vi "Create New Class or Interface in Library.vi"(6 "directory (empty)":path, 8 "error in":errorcluster, 9 "create interface":bool, 10 "new class file name":string, 11 "library reference in":refnum<vi>) -> (0 "error out":errorcluster, 2 "class reference":refnum<vi>, 3 "library reference out":refnum<vi>)   [LabVIEW 2020]
doc: "Creates a new class or interface in memory. The new class or interface is not saved to disk even if you supply a <b>directory</b>. The <b>directory</b> specifies an initial location for the class should you choose to save it to disk later. If you specify an empty directory, then the new class or interface will be assigned an initial path relative to its owning library (if any), the the current project (if any) or the LabVIEW Data directory."
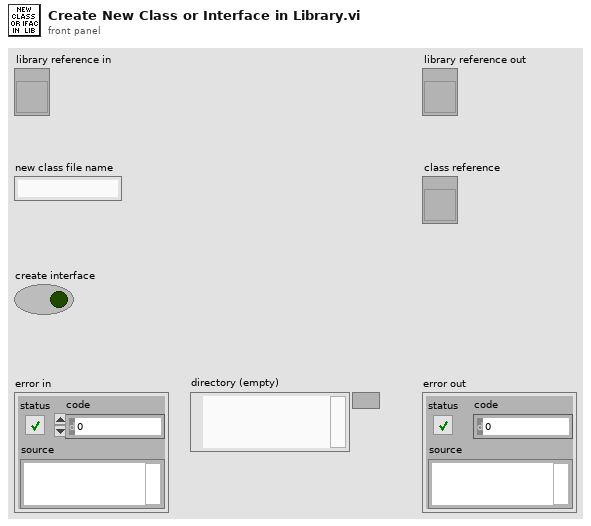
[diagram p1: front panel]
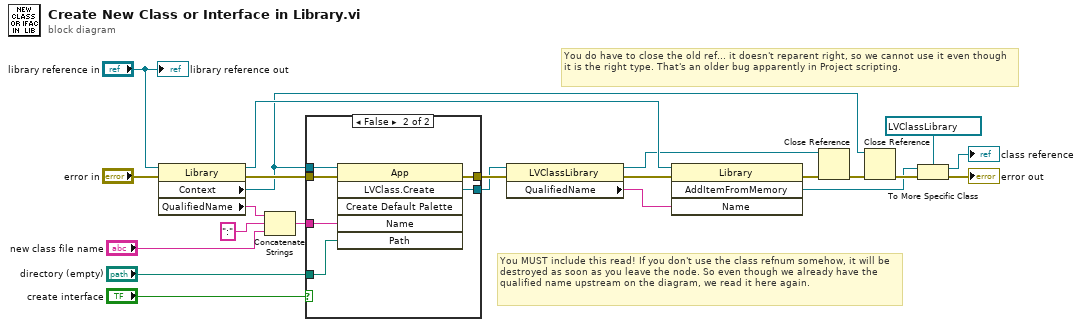
[diagram p0: block diagram]
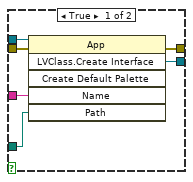
[diagram p2: hidden frame]
diagram:
  # "You do have to close the old ref... it doesn't reparent right, so we cannot use it even though it is the right type. That's an older bug apparently in Project scripting."
  # "You MUST include this read! If you don't use the class refnum somehow, it will be destroyed as soon as you leave the node. So even though we already have the qualified name upstream on the diagram, we read it here again."
  n1 = property class="Library"(reference="library reference in", error in="error in") -> (reference out=w14:refnum<vi>, error out=w23:errorcluster, "Context"=w2:refnum<vi>, "QualifiedName"=w13:string)
  n2 = Concatenate Strings(w13, ":" ("Name"), "new class file name") -> (w3:string)
  n3 = case shown="False" "create interface" {
    tunnel: w23 -> [w29 w35]
    tunnel: w3 -> [w27 w33]
    tunnel: [w26 w32] -> w12
    tunnel: [w28 w34] -> w22
    tunnel: w2 -> [w25 w30]
    tunnel: "directory (empty)" -> [w24 w31]
    frame True {
      n4 = invoke class="App" method="LVClass.Create Interface"(reference=w25, error in=w29, "Name"=w27, "Path"=w24) -> (error out=w28:errorcluster, "LVClass.Create Interface"=w26:refnum<vi>)  [unwired: 2 in, 4 out]
    }
    frame False {
      n5 = invoke class="App" method="LVClass.Create"(reference=w30, error in=w35, "Name"=w33, "Path"=w31) -> (error out=w34:errorcluster, "LVClass.Create"=w32:refnum<vi>)  [unwired: 2 in, 4 out]
    }
  }
  n6 = property class="LVClassLibrary"(reference=w12, error in=w22) -> (reference out=w10:refnum<vi>, error out=w21:errorcluster, "QualifiedName"=w1:string)
  n7 = invoke class="Library" method="AddItemFromMemory"(reference=w14, error in=w21, "Name"=w1) -> (error out=w19:errorcluster, "AddItemFromMemory"=w11:refnum<vi>)  [unwired: 1 in, 2 out]
  n8 = Close Reference(reference=w10, error in (no error)=w19) -> (error out=w17:errorcluster)
  n9 = Close Reference(reference=w2, error in (no error)=w17) -> (error out=w16:errorcluster)
  n10 = To More Specific Class(target class=refnum<vi> refnum ("reference out"), reference=w11, error in=w16) -> (specific class reference=→"class reference":refnum<vi>, error out=→"error out":errorcluster)
  "library reference out" <- "library reference in"
